vi "getcmd.vi"(4 "error in":errorcluster, 6 "srcurl":string) -> (0 "error out":errorcluster, 1 "Elements":string[](array[string]), 2 "new?":bool, 3 "lowercase file ext":string)   [LabVIEW 2010]
uses:
  <vilib>/httpClient/LabVIEWHTTPClient.lvlib
panel:
  out "XML File Path":path
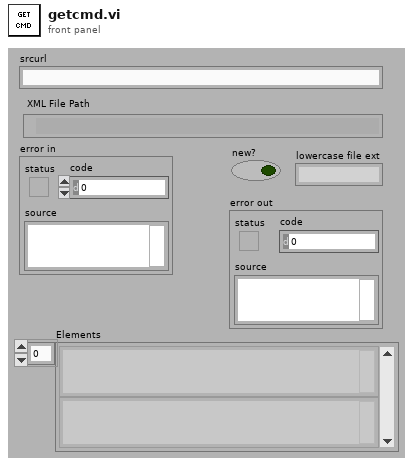
[diagram p1: front panel]
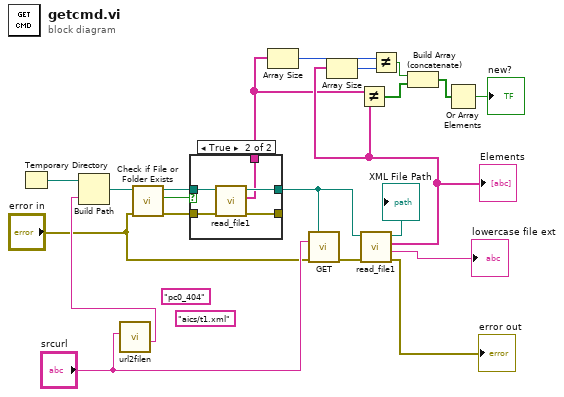
[diagram p0: block diagram]
diagram:
  (unwired) "pc0_404" ("host (this computer)")
  (unwired) "aics/t1.xml" ("virtual path")
  n1 = Temporary Directory() -> (w1:path)
  n2 = call "url2filen.vi"("srcurl"="srcurl") -> ("virtual path"=w21:string)  [unwired: 6 in]
  n3 = Build Path(base path=w1, name or relative path=w21) -> (appended path=w6:path)
  n4 = call <vilib>:"Check if File or Folder Exists.vi"("error in (no error)"="error in", "path"=w6) -> ("error out"=w8:errorcluster, "file or folder exists?"=w9:bool, "dup path"=w7:path)  [unwired: 7 in]
  n5 = case shown="True" w9 {
    tunnel: [w23 w28] -> w5
    tunnel: [_ w26] -> w11
    tunnel: w7 -> [w23 w24]
    tunnel: w8 -> [w22 w25]
    tunnel: [w22 w27] -> _
    frame False {
    }
    frame True {
      n6 = call "read_file1.vi"("error in"=w25, "file"=w24) -> ("error out"=w27:errorcluster, "Elements"=w26:string[], "File Path"=w28:path)  [unwired: 2 in, 1 out]
    }
  }
  n7 = Array Size(array=w11) -> (size(s)=w13:i32)
  n8 = call <vilib>:"GET.vi"("output file"=w5, "URL"="srcurl", "error in (no error)"="error in") -> ("error out"=w2:errorcluster)  [unwired: 9 in, 3 out]
  n9 = call "read_file1.vi"("error in"=w2, "file"=w5) -> ("error out"=→"error out":errorcluster, "lowercase file ext"=→"lowercase file ext":string, "Elements"=w12:string[], "File Path"=→"XML File Path":path)  [unwired: 2 in]
  "Elements" <- w12
  n10 = Array Size(array=w12) -> (size(s)=w14:i32)
  n11 = Not Equal?(x=w11, y=w12) -> (x != y?=w15:bool[])
  n12 = Not Equal?(x=w13, y=w14) -> (x != y?=w16:bool)
  n13 = Build Array (concatenate)(w16, w15) -> (w17:bool[])
  n14 = Or Array Elements(Boolean array=w17) -> (logical OR=→"new?":bool)
